vi "LEP_RV_UVSetCrossModuleOptimization.vi"(7 "Use Cross Module Optimization":bool, 8 "error in (no error)":errorcluster, 11 "uVision Project":path) -> (0 "error out":errorcluster)   [LabVIEW 2011]
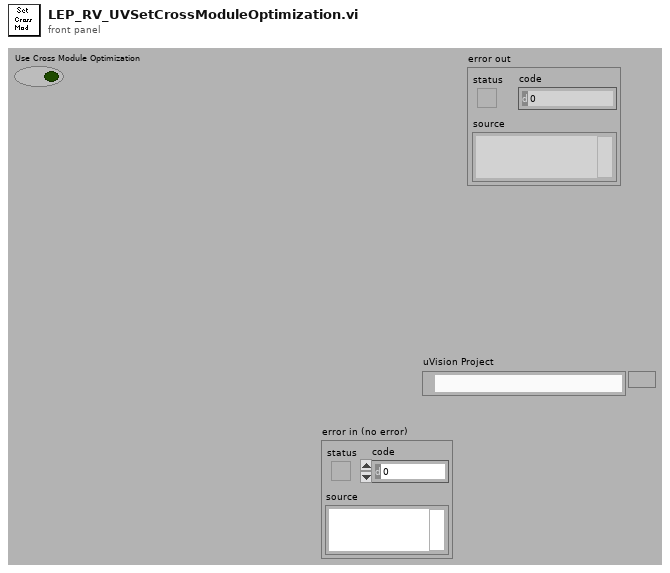
[diagram p1: front panel]
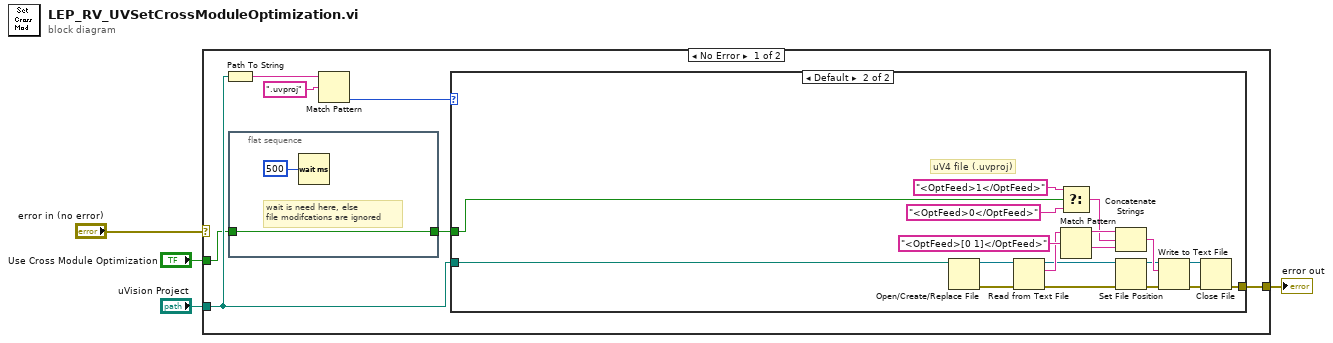
[diagram p0: block diagram]
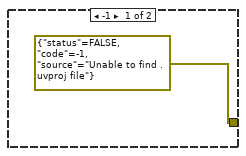
[diagram p2: hidden frame]
diagram:
  n1 = case shown="No Error" "error in (no error)" {
    selector: "error in (no error)" -> [_ w34]
    tunnel: [w7 w34] -> w3
    tunnel: "uVision Project" -> [w8 _]
    tunnel: "Use Cross Module Optimization" -> [w6 _]
    frame No Error {
      n2 = Path To String(path=w8) -> (string=w11:string)
      n3 = flat-sequence {
        tunnel: w6 -> [w12]
        tunnel: [w12] -> w5
        frame #0 {
          # "wait is need here, else\nfile modifcations are ignored"
          n4 = Wait (ms)(milliseconds to wait=u32 500) -> ()  [unwired: 1 out]
        }
      }
      n5 = Match Pattern(string=w11, regular expression=".uvproj") -> (offset past match=w9:i32)  [unwired: 1 in, 3 out]
      n6 = case shown="Default" w9 {
        tunnel: w8 -> [_ w26]
        tunnel: w5 -> [_ w30]
        tunnel: [errorcluster {"status"=FALSE, "code"=-1, "source"="Unable to find .uvproj file"} ("error out") w15] -> w7
        frame -1 {
        }
        frame Default {
          # "uV4 file (.uvproj)"
          n7 = Open/Create/Replace File(file path (use dialog)=w26) -> (refnum out=w25:refnum<file>, error out=w24:errorcluster)  [unwired: 5 in, 1 out]
          n8 = Read from Text File(file (use dialog)=w25, error in=w24) -> (refnum out=w21:refnum<file>, text=w23:string, error out=w19:errorcluster)  [unwired: 2 in, 1 out]
          n9 = Select(t="<OptFeed>1</OptFeed>", s=w30, f="<OptFeed>0</OptFeed>") -> (s? t:f=w27:string)
          n10 = Match Pattern(string=w23, regular expression="<OptFeed>[0 1]</OptFeed>") -> (before substring=w32:string, after substring=w31:string)  [unwired: 1 in, 2 out]
          n11 = Concatenate Strings(w32, w27, w31) -> (w22:string)
          n12 = Set File Position(refnum=w21, error in=w19) -> (refnum out=w20:refnum<file>, error out=w18:errorcluster)  [unwired: 2 in]
          n13 = Write to Text File(file (use dialog)=w20, text=w22, error in=w18) -> (refnum out=w17:refnum<file>, error out=w16:errorcluster)  [unwired: 1 in, 1 out]
          n14 = Close File(refnum=w17, error in=w16) -> (error out=w15:errorcluster)  [unwired: 1 out]
        }
      }
    }
    frame Error {
    }
  }
  "error out" <- w3
